vi "1420serial.vi"() -> ()   [LabVIEW 2019]
doc: "This example sets the RS-485 transceiver control modes for the specified port and performs a serial port read, a serial port write, or a combination of these actions. If all are selected, the VI will write the data first, read data and then close the VISA session that is opened to the port. This VI will wait until the specified number of bytes is received at the port or until a termination character is received. This example will work only with National Instruments RS-485 interfaces.\n\nThis example demonstrates the transceiver control modes available when using a National Instruments RS-485 product. When connecting one or several devices via RS-485, a user may want to cut down on the amount of wiring. Alternatively, some devices offer a certain wiring configuration that you may need to match. Determine the wiring needs of the connected serial device to determine which NI RS-485 transceiver control mode to choose.\n\nWhen you are communicating with a two-wire device, National Instruments recommends that you use the two-wire Auto Control mode. This mode handles the transmitter/receiver enabling for a two-wire connection in your hardware, so it reduces the software overhead required to perform this operation in your application program."
uses:
  Program Files (x86)/National Instruments/LabVIEW 2019/examples/Instrument IO/Serial/support/Serial - Settings.ctl
panel:
  out "x*y":dbl
  in  "stop":bool
  in  "Termination Character":u8=10 format="%.0x"
  in  "End Write on Termination Character?":bool=TRUE
  in  "End Read on Termination Character?":bool=TRUE
  in  "Write String":string="*IDN?"
  in  "Serial Settings":T1={"baud rate"=9600, "data bits"=8, "parity"=enum."None", "stop bits"=10, "flow control"=0} {"flow control" items=["None"=0, "XON/XOFF"=1, "RTS/CTS"=2, "DTR/DSR"=4]; "stop bits" items=["1.0"=10, "1.5"=15, "2.0"=20]; "data bits" min=5 max=8 step=1; "baud rate" items=["75"=75, "110"=110, "134"=134, "150"=150, "300"=300, "600"=600, "1200"=1200, "1800"=1800, "2400"=2400, "4800"=4800, "7200"=7200, "9600"=9600, "14400"=14400, "19200"=19200, "28800"=28800, "38400"=38400, "56000"=56000, "57600"=57600, "115200"=115200, "128000"=128000, "230400"=230400]}
  in  "Assert DTR?":bool
  in  "VISA RS 485 Resource":refnum<visa-resource-name>="COM1"
  # "Overview: Demonstrates the use of the VISA functions to configure NI RS-485 hardware.\nRequirements: NI-Serial and NI-VISA Drivers, NI RS-485 hardware\nInstructions:\n1. Ensure the resource specified in the VISA RS 485 Resource control is a valid NI RS-485 device, and that the Assert DTR? value is correct for your device.\n2. Specify the proper RS-485 Transceiver Mode value for your device.\n3. Run the VI.\n4. View the Response returned by the device."
  # "0xA is equivalent to a '\\n' character, which is a line feed."
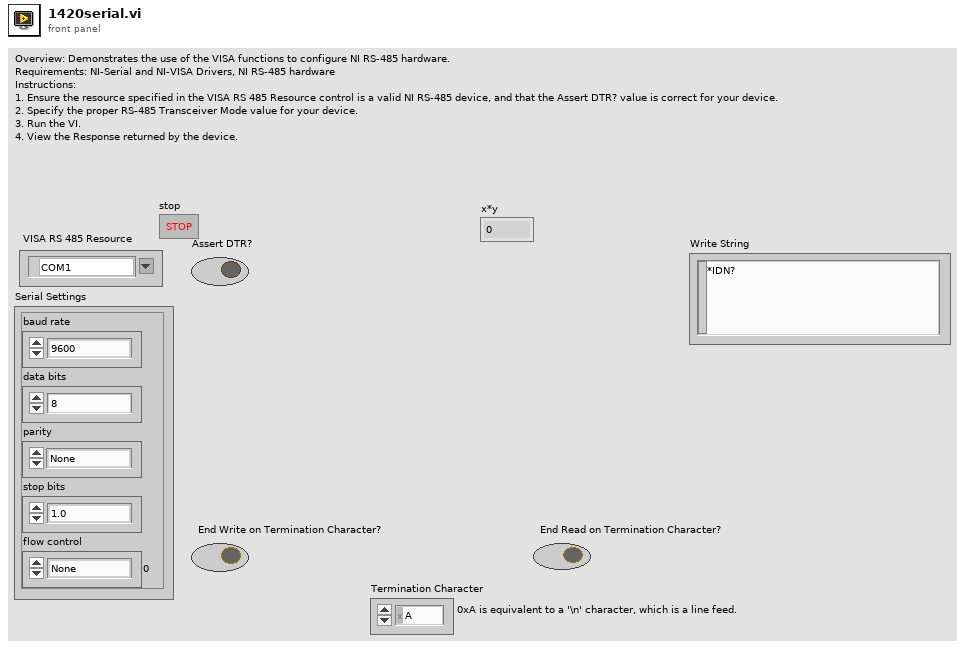
[diagram p1: front panel]
types:
  T1 = typedef "Serial - Settings.ctl" = cluster{"baud rate":u32, "data bits":u16, "parity":enum16{"None", "Odd", "Even", "Mark", "Space"}, "stop bits":u16, "flow control":u16}
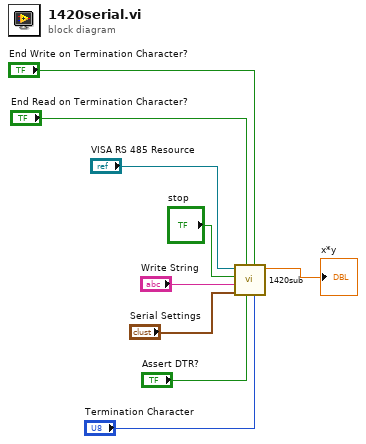
[diagram p0: block diagram]
diagram:
  n1 = call "1420sub.vi"("Termination Character"="Termination Character", "End Write on Termination Character?"="End Write on Termination Character?", "Assert DTR?"="Assert DTR?", "End Read on Termination Character?"="End Read on Termination Character?", "Serial Settings"="Serial Settings", "Write String"="Write String", "stop"="stop", "VISA Refnum in"="VISA RS 485 Resource") -> ("x*y"=→"x*y":dbl)  [unwired: 3 in]
